vi "Pre Launch Init.vi"(11 "Counter in":refnum<class "Counter.lvclass">) -> (0 "error out":errorcluster, 3 "Counter out":refnum<class "Counter.lvclass">)   [LabVIEW 2018, in "Counter.lvlib" / "Counter.lvclass"]
doc: "(<B>Filename</B>: Actor Framework.lvlib:Actor.lvclass:Pre Launch Init.vi)\n\nDefines behavior that occurs after the Launch Nested Actor method is invoked but before the actor's Actor Core method begins running.\n\nBy default, this method does nothing. A descendant class may override it to define behavior."
uses:
  Counter.lvclass
  Counter.lvclass/Counter.ctl
  <vilib>/ActorFramework/Actor/Actor.lvclass
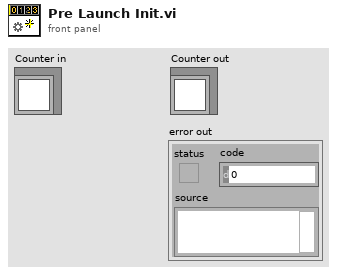
[diagram p1: front panel]
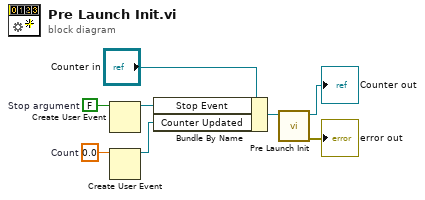
[diagram p0: block diagram]
diagram:
  w2 = 0.0  # Count
  w4 = FALSE  # Stop argument
  n1 = Create User Event(user event datatype=w4) -> (user event=w3:refnum<user-event>)  [unwired: 1 in, 1 out]
  n2 = Create User Event(user event datatype=w2) -> (user event=w1:refnum<user-event>)  [unwired: 1 in, 1 out]
  n3 = Bundle By Name(cluster="Counter in", "Stop Event"=w3, "Counter Updated"=w1) -> (w5:refnum<class "Counter.lvclass">)
  n4 = call-parent "Pre Launch Init.vi"("Actor in"=w5) -> ("error out"=→"error out":errorcluster, "Actor out"=→"Counter out":refnum<class "Counter.lvclass">)  [unwired: 9 in]
